vi "destroySubDataEvents.vi"(8 "error in (no error)":errorcluster, 11 "DataListenerThisComponent in":refnum<class "DataListenerThisComponent.lvclass">) -> (0 "error out":errorcluster, 3 "DataListenerThisComponent out":refnum<class "DataListenerThisComponent.lvclass">)   [LabVIEW 2015]
uses:
  DataListenerThisComponent.lvclass
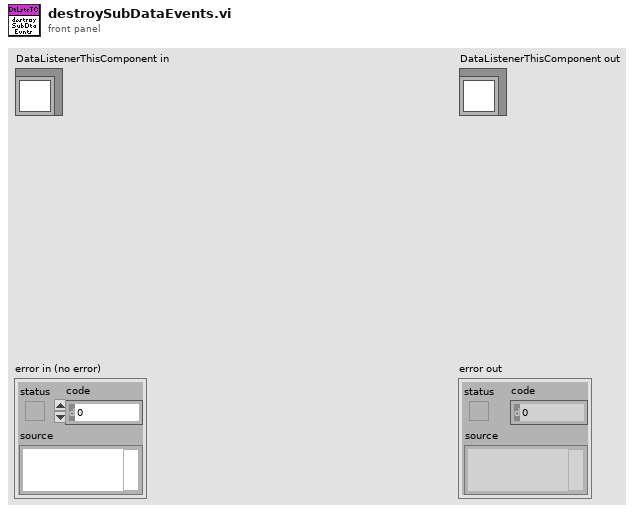
[diagram p1: front panel]
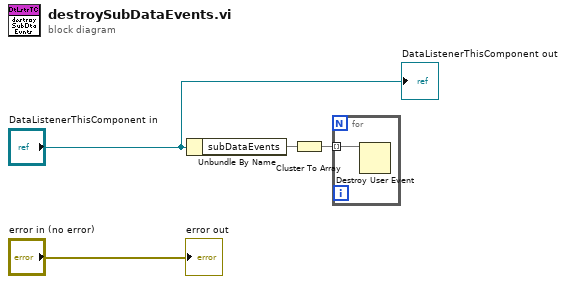
[diagram p0: block diagram]
diagram:
  n1 = Unbundle By Name("DataListenerThisComponent in") -> ("subDataEvents"=w2)
  n2 = Cluster To Array(cluster=w2) -> (array=w3:void[])
  n3 = for {
    tunnel: w3 -> [w5] mode=indexing
    n4 = Destroy User Event(user event=w5) -> ()  [unwired: 1 in, 1 out]
  }
  "error out" <- "error in (no error)"
  "DataListenerThisComponent out" <- "DataListenerThisComponent in"
